vi "TPNT_SendCommand.vi"(4 "error in (no error)":errorcluster, 5 "inmediate reply Timeout ms (5000)":i32=5000, 6 "ReplyQ":string, 7 "Command":string) -> (0 "error out":errorcluster, 1 "Reply":string)   [LabVIEW 2016]
doc: "This VI sends generic commands to the Modules Manager Module. The list of available commands is under the MDMGR_Main.vi description"
panel:
  in  "CmdStruct":cluster{"command":string, "respondTo":string}
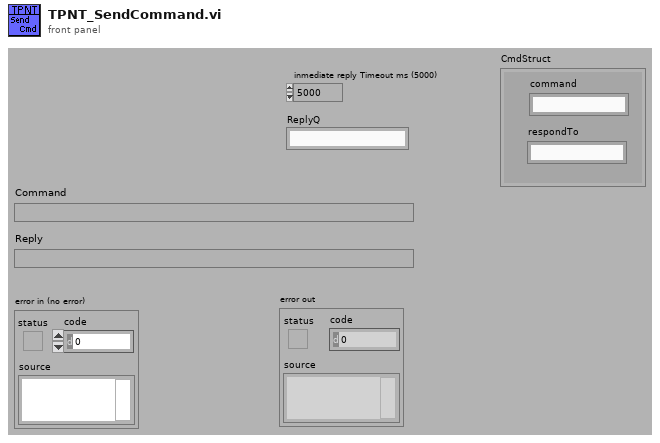
[diagram p1: front panel]
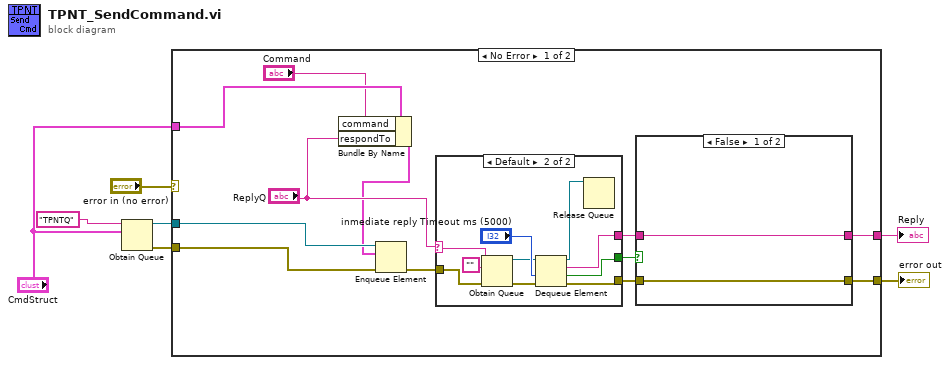
[diagram p0: block diagram]
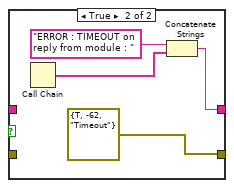
[diagram p2: hidden frame]
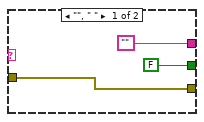
[diagram p3: hidden frame]
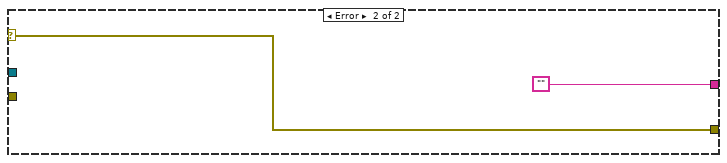
[diagram p4: hidden frame]
diagram:
  n1 = Obtain Queue(name (unnamed)="TPNTQ", element data type="CmdStruct") -> (queue out=w3:refnum<queue>, error out=w2:errorcluster)  [unwired: 3 in, 1 out]
  n2 = case shown="No Error" "error in (no error)" {
    selector: "error in (no error)" -> [_ w40]
    tunnel: [w15 w40] -> w6
    tunnel: [w17 ""] -> w5
    tunnel: w3 -> [w14 _]
    tunnel: w2 -> [w13 _]
    tunnel: "CmdStruct" -> [w9 _]
    frame No Error {
      n3 = Bundle By Name(cluster=w9, "command"="Command", "respondTo"="ReplyQ") -> (w10:cluster{"command":string, "respondTo":string})
      n4 = Enqueue Element(queue=w14, element=w10, error in (no error)=w13) -> (error out=w12:errorcluster)  [unwired: 3 out]
      n5 = case shown="Default" "ReplyQ" {
        selector: "ReplyQ" -> [_ w38]
        tunnel: [w26 w36] -> w16
        tunnel: ["" ("queue element") w31] -> w18
        tunnel: [FALSE ("timed out") w32] -> w19
        tunnel: w12 -> [w26 w29]
        frame "", " " {
        }
        frame Default {
          n6 = Obtain Queue(name (unnamed)=w38, element data type="", error in (no error)=w29) -> (queue out=w34:refnum<queue>, error out=w33:errorcluster)  [unwired: 2 in, 1 out]
          n7 = Dequeue Element(queue=w34, timeout in ms (-1)="inmediate reply Timeout ms (5000)", error in (no error)=w33) -> (queue out=w30:refnum<queue>, element=w31:string, timed out?=w32:bool, error out=w36:errorcluster)
          n8 = Release Queue(queue=w30) -> ()  [unwired: 1 in, 4 out]
        }
      }
      n9 = case shown="False" w19 {
        tunnel: [w21 w25] -> w17
        tunnel: w18 -> [w21 _]
        tunnel: w16 -> [w20 _]
        tunnel: [w20 errorcluster {"status"=TRUE, "code"=-62, "source"="Timeout"} ("error out")] -> w15
        frame False {
        }
        frame True {
          n10 = Call Chain() -> (call chain=w23:string[])
          n11 = Concatenate Strings("ERROR : TIMEOUT on reply from module : ", w23) -> (w25:string)
        }
      }
    }
    frame Error {
    }
  }
  "error out" <- w6
  "Reply" <- w5
